vi "Begin.vi"(8 "error in":errorcluster) -> (0 "error out":errorcluster)   [LabVIEW 2014]
doc: "Called before other user functions, this VI is expected to open initial I/O refnums, load in file data, and do all program initialization. Notice that the <B>error out</B> terminal is simply used for data flow. Wiring it to other structures or subVIs ensures that this VI runs first."
uses:
  <vilib>/Rock Robotics/WPI/DriverStation/WPI_DriverStationRobotMode2.ctl
  <vilib>/Rock Robotics/WPI/Joystick/WPI_JoystickDeviceEnum.ctl
  <vilib>/Rock Robotics/SystemInterfaces/DIO/FPGA_DIOChannel.ctl
  <vilib>/Rock Robotics/WPI/Solenoid/WPI_SolenoidChannel.ctl
  <vilib>/Rock Robotics/WPI/SafetyOutput/WPI_SafetyOutputConfigMenu.ctl
  <vilib>/Rock Robotics/SystemInterfaces/DIO/FPGA_DIOPWMChannel.ctl
  Robot Global Data.vi
  <vilib>/Rock Robotics/Network Tables/SD Write String Array.vi
  <vilib>/Rock Robotics/WPI/Switch/WPI_SwitchOpenLimit.vi
  <vilib>/Rock Robotics/WPI/Ultrasonic/WPI_SonarSRF04DigitalOpen.vi
  <vilib>/Rock Robotics/WPI/Ultrasonic/WPI_SonarSRF04DigitalRefNum Registry Set.vi
  <vilib>/Rock Robotics/WPI/Solenoid/WPI_SolenoidOpenSingle.vi
  <vilib>/Rock Robotics/WPI/MotorControl/WPI_MotorControlOpenCANTalonSRX.vi
  <vilib>/Rock Robotics/WPI/MotorControl/WPI_MotorControlOpen Talon.vi
  <vilib>/Rock Robotics/WPI/Accelerometer/InternalAccelerometer/WPI_AccelerometerInternalOpen.vi
  <vilib>/Rock Robotics/WPI/RobotDrive/WPI_RobotDriveOpen4MotorWithCANTalonSRX.vi
  <vilib>/NI/AMC/AMC.lvlib
  <vilib>/Rock Robotics/WPI/RobotDrive/WPI_RobotDriveOpen4MotorWithTalon.vi
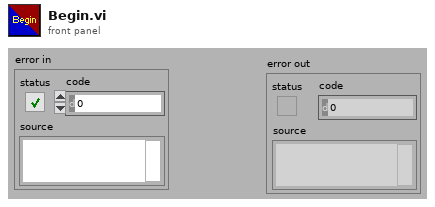
[diagram p1: front panel]
types:
  T1 = typedef "FPGA_DIOChannel.ctl" = enum8{"DIO 0", "DIO 1", "DIO 2", "DIO 3", "DIO 4", "DIO 5", "DIO 6", "DIO 7", "DIO 8", "DIO 9", "DIO MXP 0", "DIO MXP 1", "DIO MXP 2", "DIO MXP 3", "DIO MXP 4", "DIO MXP 5", "DIO MXP 6", "DIO MXP 7", "DIO MXP 8", "DIO MXP 9", "DIO MXP 10", "DIO MXP 11", "DIO MXP 12", "DIO MXP 13", "DIO MXP 14", "DIO MXP 15", "Invalid"}
  T2 = typedef "FPGA_DIOPWMChannel.ctl" = enum8{"PWM 0", "PWM 1", "PWM 2", "PWM 3", "PWM 4", "PWM 5", "PWM 6", "PWM 7", "PWM 8", "PWM 9", "PWM MXP 0", "PWM MXP 1", "PWM MXP 2", "PWM MXP 3", "PWM MXP 4", "PWM MXP 5", "PWM MXP 6", "PWM MXP 7", "PWM MXP 8", "PWM MXP 9", "Invalid"}
  T3 = typedef "WPI_SafetyOutputConfigMenu.ctl" = enum16{"Enable", "Disable"}
  T4 = typedef "WPI_SolenoidChannel.ctl" = enum8{"Solenoid 0", "Solenoid 1", "Solenoid 2", "Solenoid 3", "Solenoid 4", "Solenoid 5", "Solenoid 6", "Solenoid 7", "Invalid"}
  T5 = typedef "WPI_JoystickDeviceEnum.ctl" = enum16{"USB 0", "USB 1", "USB 2", "USB 3", "USB 4", "USB 5"}
  T6 = typedef "WPI_DriverStationRobotMode2.ctl" = enum16{"Autonomous Disabled", "Autonomous Enabled", "Teleop Disabled", "Teleop Enabled", "Disconnected", "Finish", "Test Disabled", "Test Enabled", "Emergency Stopped"}
  T7 = typedef "WPI_RobotDriveDevRef.ctl" = cluster{"DevStatus":errorcluster, "Motors[]":T8[], "Square Inputs":bool, "Max Output":dbl}
  T8 = typedef "WPI_MotorControlDeviceRef.ctl" = cluster{"DeviceStatus":errorcluster, "Type":T9, "PWM":cluster{"Controller":T10, "PWM Channel":T2, "DeadBand":T11}, "CAN":cluster{"Device Number":u8, "Control Mode":T12, "Semaphore":T13, "Max Vout":dbl, "TalonSRX Control Mode":T14}, "Invert":bool, "TransformRef":T15, "InvTransformRef":T15}
  T9 = typedef "WPI_MotorControlType.ctl" = enum16{"PWM", "CAN", "CANTalonSRX"}
  T10 = typedef "FPGA_TypedefDigitalModule.ctl" = enum16{"Controller 1"}
  T11 = typedef "WPI_PWMDeadband.ctl" = cluster{"Name":string, "maxPositivePwm":i32, "minPositivePwm":i32, "centerPwm":i32, "maxNegativePwm":i32, "minNegativePwm":i32, "angularRange":u16}
  T12 = typedef "WPI_CANJaguar_ControlMode.ctl" = enum8{"Percent VBus", "Current", "Speed", "Position", "Voltage"}
  T13 = typedef "Semaphore RefNum" = refnum<k1>
  T14 = typedef "WPI_CANTalonSRX_APIControlMode.ctl" = enum8{"Percent VBus", "Speed", "Position", "Slave", "Unchanged / Invalid"}
  T15 = typedef "WPI_PWMTransform_ConPane.ctl" = refnum<vi>
  T16 = typedef "WPI_JoystickDevRef.ctl" = cluster{"Device":T5}
  T17 = typedef "WPI_SolenoidDevRef.ctl" = cluster{"DevStatus":errorcluster, "Pneumatics Control Module":u8, "Forward Solenoid Channel":T4, "Reverse Solenoid Channel":T4}
  T18 = typedef "WPI_AccelerometerDevRef.ctl" = cluster{"DevStatus":errorcluster, "Controller":T19, "Scaling":T20, "Analog Channels":T21, "I2C Bus":T23, "SPI Bus":T24, "Accel Range":T25, "ADXL345 Axes":T26, "Handle":i32, "Device Address":u8, "Accel Type":enum16{"Analog", "ADXL345 I2C", "ADXL345 SPI", "Internal"}}
  T19 = typedef "FPGA_TypedefAnalogModule.ctl" = enum16{"Controller 1"}
  T20 = typedef "WPI_AccelerometerScaling.ctl" = cluster{"Gain (VoltsPerG)":dbl, "Center Voltage":dbl}
  T21 = typedef "WPI_AccelerometerAnalogChannels.ctl" = cluster{"X-Axis":T22, "Y-Axis":T22, "Z-Axis":T22}
  T22 = typedef "FPGA_AIChannel.ctl" = enum8{"AI 0", "AI 1", "AI 2", "AI 3", "AI MXP 0", "AI MXP 1", "AI MXP 2", "AI MXP 3", "Invalid"}
  T23 = typedef "i2c_bus.ctl" = enum16{"I2C On-Board", "I2C MXP", "Invalid"}
  T24 = typedef "spi_bus.ctl" = enum16{"SPI On-Board, CS0", "SPI On-Board, CS1", "SPI On-Board, CS2", "SPI On-Board, CS3", "SPI MXP", "Invalid"}
  T25 = typedef "ADXL345 Range.ctl" = u8
  T26 = typedef "WPI_AccelerometerADXL345 Axes.ctl" = cluster{"X-Axis":bool, "Y-Axis":bool, "Z-Axis":bool}
  T27 = typedef "WPI_SwitchDevRef.ctl" = cluster{"DevStatus":errorcluster, "DIO Channel":T1, "Controller":T10, "CntIndex":T28, "Normally Closed":bool}
  T28 = typedef "FPGA_CounterCtrSystemIndex.ctl" = enum8{"Ctr 0", "Ctr 1", "Ctr 2", "Ctr 3", "Ctr 4", "Ctr 5", "Ctr 6", "Ctr 7", "Invalid"}
  T29 = typedef "WPI_UltrasonicDeviceRef.ctl" = cluster{"DevStatus":errorcluster, "Ping Digital Controller":T10, "Echo Digital Controller":T10, "Ping Channel":T1, "Echo Channel":T1, "CntIndex":T28}
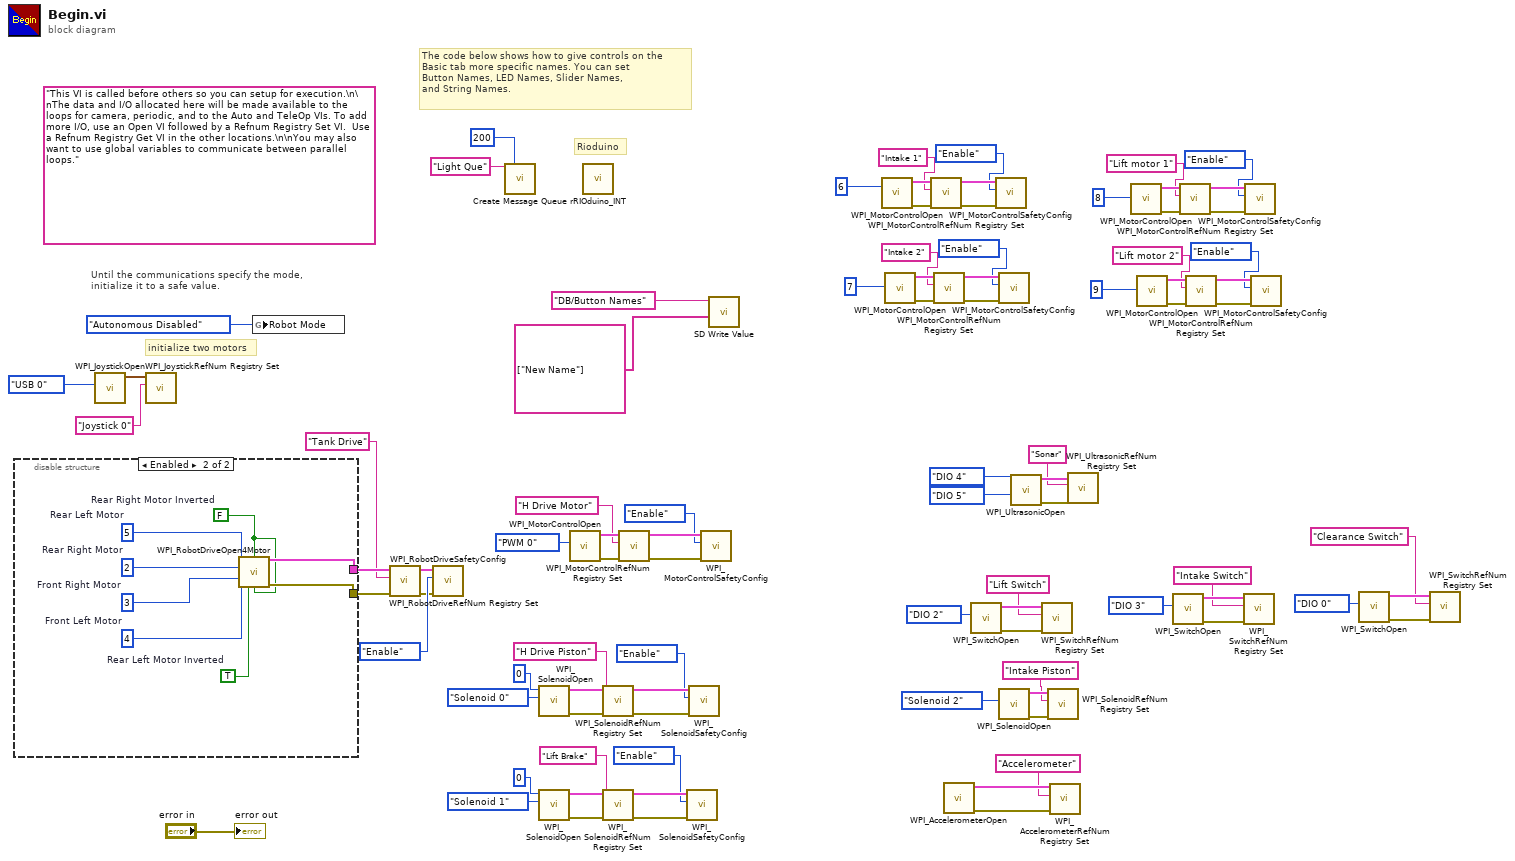
[diagram p0: block diagram]
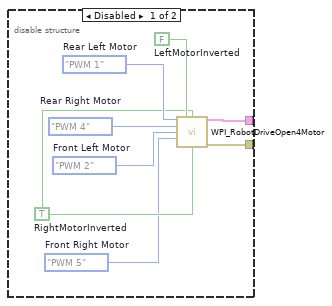
[diagram p2: hidden frame]
diagram:
  (unwired) "This VI is called before others so you can setup for execution.\n\nThe data and I/O allocated here will be made available to the loops for camera, periodic, and to the Auto and TeleOp VIs. To add more I/O, use an Open VI followed by a Refnum Registry Set VI.  Use a Refnum Registry Get VI in the other locations.\n\nYou may also want to use global variables to communicate between parallel loops."
  # "Rioduino"
  # "The code below shows how to give controls on the\nBasic tab more specific names. You can set\nButton Names, LED Names, Slider Names,\nand String Names."
  # "Until the communications specify the mode,\ninitialize it to a safe value."
  # "initialize two motors"
  n1 = disable-structure shown="Enabled" {
    disable-tunnel: [w98 w106] -> w41
    disable-tunnel: [w97 w105] -> w40
    frame Disabled {
      w91 = FPGA_DIOPWMChannel."PWM 5"  # Front Right Motor
      w92 = TRUE  # RightMotorInverted
      w93 = FPGA_DIOPWMChannel."PWM 1"  # Rear Left Motor
      w94 = FALSE  # LeftMotorInverted
      w95 = FPGA_DIOPWMChannel."PWM 2"  # Front Left Motor
      w96 = FPGA_DIOPWMChannel."PWM 4"  # Rear Right Motor
      n2 = call-poly <vilib>:"WPI_RobotDriveOpen4Motor.vi"("Rear Left Motor"=w93, "Rear Left Motor Inverted"=w94, "Rear Right Motor Inverted"=w92, "Rear Right Motor"=w96, "Front Left Motor"=w95, "Front Right Motor"=w91, "Front Right Motor Inverted"=w92) -> ("RobotDriveDevRef"=w98:T7, "error out"=w97:errorcluster)  [unwired: 7 in]
    }
    frame Enabled {
      w99 = u8 3  # Front Right Motor
      w100 = u8 4  # Front Left Motor
      w101 = u8 2  # Rear Right Motor
      w102 = TRUE  # Rear Left Motor Inverted
      w103 = FALSE  # Rear Right Motor Inverted
      w104 = u8 5  # Rear Left Motor
      n3 = call-poly <vilib>:"WPI_RobotDriveOpen4Motor.vi"("Rear Left Motor"=w104, "Rear Left Motor Inverted"=w102, "Rear Right Motor Inverted"=w103, "Rear Right Motor"=w101, "Front Left Motor"=w100, "Front Right Motor"=w99, "Front Left Motor Inverted"=w102, "Front Right Motor Inverted"=w103) -> ("RobotDriveDevRef"=w106:T7, "error out"=w105:errorcluster)  [unwired: 6 in]
    }
  }
  n4 = call <vilib>:"WPI_JoystickOpen.vi"("JoystickDevice"=WPI_JoystickDeviceEnum."USB 0") -> ("JoystickDevRef"=w86:T16)  [unwired: 10 in]
  n5 = call <vilib>:"WPI_JoystickRefNum Registry Set.vi"("refnum name"="Joystick 0", "JoystickDevRef"=w86) -> ()  [unwired: 8 in, 2 out]
  n6 = global write "Robot Global Data.vi" "Robot Mode"(WPI_DriverStationRobotMode2."Autonomous Disabled" ("Robot Mode")) -> ()
  n7 = call <vilib>:"WPI_RobotDriveRefNum Registry Set.vi"("error in (no error)"=w40, "refnum name"="Tank Drive", "RobotDriveDevRef"=w41) -> ("error out"=w10:errorcluster, "RobotDriveDevRef"=w90:T7)  [unwired: 7 out]
  n8 = call <vilib>:"WPI_RobotDriveSafetyConfig.vi"("error in (no error)"=w10, "mode"=WPI_SafetyOutputConfigMenu."Enable", "RobotDriveDevRef"=w90) -> ()  [unwired: 7 in, 2 out]
  n9 = call <vilib>:"Create Message Queue.vi"("message queue name"="Light Que", "max queue size (-1, unlimited)"=200) -> ()  [unwired: 12 in, 2 out]
  n10 = call-poly <vilib>:"WPI_SolenoidOpen.vi"("Solenoid Channel"=WPI_SolenoidChannel."Solenoid 0", "Pneumatics Control Module (0)"=u8 0) -> ("error out"=w28:errorcluster, "SolenoidDevRef"=w29:T17)  [unwired: 8 in]
  n11 = call-poly <vilib>:"WPI_SolenoidOpen.vi"("Solenoid Channel"=WPI_SolenoidChannel."Solenoid 1", "Pneumatics Control Module (0)"=u8 0) -> ("error out"=w25:errorcluster, "SolenoidDevRef"=w24:T17)  [unwired: 8 in]
  n12 = call-poly <vilib>:"WPI_MotorControlOpen.vi"("PWM Channel"=FPGA_DIOPWMChannel."PWM 0") -> ("error out"=w39:errorcluster, "MotorControlDeviceRef"=w38:T8)  [unwired: 9 in]
  n13 = call "rRIOduino_INT.vi"() -> ()  [unwired: 12 in]
  n14 = call <vilib>:"WPI_SolenoidRefNum Registry Set.vi"("error in (no error)"=w28, "refnum name"="H Drive Piston", "SolenoidDevRef"=w29) -> ("error out"=w20:errorcluster, "SolenoidDevRef"=w21:T17)  [unwired: 7 in]
  n15 = call <vilib>:"WPI_SolenoidRefNum Registry Set.vi"("error in (no error)"=w25, "refnum name"="Lift Brake", "SolenoidDevRef"=w24) -> ("error out"=w19:errorcluster, "SolenoidDevRef"=w18:T17)  [unwired: 7 in]
  n16 = call <vilib>:"WPI_MotorControlRefNum Registry Set.vi"("error in (no error)"=w39, "refnum name"="H Drive Motor", "MotorControlDevRef"=w38) -> ("error out"=w37:errorcluster, "MotorControlDevRef"=w36:T8)  [unwired: 7 in]
  n17 = call <vilib>:"WPI_SolenoidSafetyConfig.vi"("error in (no error)"=w19, "mode"=WPI_SafetyOutputConfigMenu."Enable", "SolenoidDevRef"=w18) -> ()  [unwired: 7 in, 2 out]
  n18 = call <vilib>:"WPI_SolenoidSafetyConfig.vi"("error in (no error)"=w20, "mode"=WPI_SafetyOutputConfigMenu."Enable", "SolenoidDevRef"=w21) -> ()  [unwired: 7 in, 2 out]
  n19 = call <vilib>:"WPI_MotorControlSafetyConfig.vi"("error in (no error)"=w37, "mode"=WPI_SafetyOutputConfigMenu."Enable", "MotorControlDevRef"=w36) -> ()  [unwired: 7 in, 2 out]
  n20 = call-poly <vilib>:"SD Write Value.vi"("String Array"=string[] ["New Name"], "Name"="DB/Button Names") -> ()  [unwired: 8 in, 2 out]
  n21 = call-poly <vilib>:"WPI_MotorControlOpen.vi"("Device Number"=u8 6) -> ("error out"=w75:errorcluster, "MotorControlDeviceRef"=w74:T8)  [unwired: 9 in]
  n22 = call-poly <vilib>:"WPI_MotorControlOpen.vi"("Device Number"=u8 7) -> ("error out"=w58:errorcluster, "MotorControlDeviceRef"=w57:T8)  [unwired: 9 in]
  n23 = call <vilib>:"WPI_MotorControlRefNum Registry Set.vi"("error in (no error)"=w75, "refnum name"="Intake 1", "MotorControlDevRef"=w74) -> ("error out"=w77:errorcluster, "MotorControlDevRef"=w76:T8)  [unwired: 7 in]
  n24 = call <vilib>:"WPI_MotorControlRefNum Registry Set.vi"("error in (no error)"=w58, "refnum name"="Intake 2", "MotorControlDevRef"=w57) -> ("error out"=w60:errorcluster, "MotorControlDevRef"=w59:T8)  [unwired: 7 in]
  n25 = call-poly <vilib>:"WPI_AccelerometerOpen.vi"() -> ("error out"=w50:errorcluster, "AccelerometerDevRef"=w49:T18)  [unwired: 10 in]
  n26 = call-poly <vilib>:"WPI_SwitchOpen.vi"("DIO Channel"=FPGA_DIOChannel."DIO 2") -> ("error out"=w71:errorcluster, "SwitchDevRef"=w70:T27)  [unwired: 9 in]
  n27 = call <vilib>:"WPI_MotorControlSafetyConfig.vi"("error in (no error)"=w77, "mode"=WPI_SafetyOutputConfigMenu."Enable", "MotorControlDevRef"=w76) -> ()  [unwired: 7 in, 2 out]
  n28 = call <vilib>:"WPI_MotorControlSafetyConfig.vi"("error in (no error)"=w60, "mode"=WPI_SafetyOutputConfigMenu."Enable", "MotorControlDevRef"=w59) -> ()  [unwired: 7 in, 2 out]
  n29 = call-poly <vilib>:"WPI_SolenoidOpen.vi"("Solenoid Channel"=WPI_SolenoidChannel."Solenoid 2") -> ("error out"=w54:errorcluster, "SolenoidDevRef"=w53:T17)  [unwired: 9 in]
  n30 = call-poly <vilib>:"WPI_UltrasonicOpen.vi"("Echo DIO Channel"=FPGA_DIOChannel."DIO 5", "Ping DIO Channel"=FPGA_DIOChannel."DIO 4") -> ("error out"=w67:errorcluster, "SonarSRF04DevRef"=w66:T29)  [unwired: 8 in]
  n31 = call <vilib>:"WPI_SwitchRefNum Registry Set.vi"("error in (no error)"=w71, "refnum name"="Lift Switch", "SwitchDevRef"=w70) -> ()  [unwired: 7 in, 2 out]
  n32 = call <vilib>:"WPI_SolenoidRefNum Registry Set.vi"("error in (no error)"=w54, "refnum name"="Intake Piston", "SolenoidDevRef"=w53) -> ()  [unwired: 7 in, 2 out]
  n33 = call <vilib>:"WPI_AccelerometerRefNum Registry Set.vi"("error in (no error)"=w50, "refnum name"="Accelerometer", "AccelerometerDevRef"=w49) -> ()  [unwired: 7 in, 2 out]
  n34 = call-poly <vilib>:"WPI_UltrasonicRefNum Registry Set.vi"("error in (no error)"=w67, "refnum name"="Sonar", "SonarSRF04DevRef"=w66) -> ()  [unwired: 7 in, 2 out]
  n35 = call-poly <vilib>:"WPI_MotorControlOpen.vi"("Device Number"=u8 8) -> ("error out"=w45:errorcluster, "MotorControlDeviceRef"=w44:T8)  [unwired: 9 in]
  n36 = call-poly <vilib>:"WPI_MotorControlOpen.vi"("Device Number"=u8 9) -> ("error out"=w81:errorcluster, "MotorControlDeviceRef"=w80:T8)  [unwired: 9 in]
  n37 = call-poly <vilib>:"WPI_SwitchOpen.vi"("DIO Channel"=FPGA_DIOChannel."DIO 3") -> ("error out"=w15:errorcluster, "SwitchDevRef"=w14:T27)  [unwired: 9 in]
  n38 = call <vilib>:"WPI_MotorControlRefNum Registry Set.vi"("error in (no error)"=w45, "refnum name"="Lift motor 1", "MotorControlDevRef"=w44) -> ("error out"=w47:errorcluster, "MotorControlDevRef"=w46:T8)  [unwired: 7 in]
  n39 = call <vilib>:"WPI_MotorControlRefNum Registry Set.vi"("error in (no error)"=w81, "refnum name"="Lift motor 2", "MotorControlDevRef"=w80) -> ("error out"=w83:errorcluster, "MotorControlDevRef"=w82:T8)  [unwired: 7 in]
  n40 = call <vilib>:"WPI_SwitchRefNum Registry Set.vi"("error in (no error)"=w15, "refnum name"="Intake Switch", "SwitchDevRef"=w14) -> ()  [unwired: 7 in, 2 out]
  n41 = call <vilib>:"WPI_MotorControlSafetyConfig.vi"("error in (no error)"=w47, "mode"=WPI_SafetyOutputConfigMenu."Enable", "MotorControlDevRef"=w46) -> ()  [unwired: 7 in, 2 out]
  n42 = call <vilib>:"WPI_MotorControlSafetyConfig.vi"("error in (no error)"=w83, "mode"=WPI_SafetyOutputConfigMenu."Enable", "MotorControlDevRef"=w82) -> ()  [unwired: 7 in, 2 out]
  n43 = call-poly <vilib>:"WPI_SwitchOpen.vi"("DIO Channel"=FPGA_DIOChannel."DIO 0") -> ("error out"=w2:errorcluster, "SwitchDevRef"=w3:T27)  [unwired: 9 in]
  n44 = call <vilib>:"WPI_SwitchRefNum Registry Set.vi"("error in (no error)"=w2, "refnum name"="Clearance Switch", "SwitchDevRef"=w3) -> ()  [unwired: 7 in, 2 out]
  "error out" <- "error in"
